vi "Terminate.vi"(8 "error in (no error)":errorcluster, 10 "Message in":refnum<class "TerminateMessage.lvclass">, 11 "DAQCascade512 in":refnum<class "DAQCascade512.lvclass">) -> (0 "error out":errorcluster, 3 "DAQCascade512 out":refnum<class "DAQCascade512.lvclass">)   [LabVIEW 2012, in "DAQCascade512.lvclass"]
doc: "This member function is called when the statemachine in the run.vi receives an 'terminate' command. It closes the RabbitMQ connection. \n\nOverride this member function in your derived class to release all previously acquired resources (but don't forget to call the parent method). If your component has subcomponents, they count as resources, and you have to release them by calling their own terminate functions."
uses:
  DAQCascade512.lvclass
  <vilib>/Distrio/Murmex/TerminateMessage/TerminateMessage.lvclass
  <vilib>/Distrio/Murmex/Murmex/Murmex.lvclass
  DAQCascade512.lvclass/DAQCascade512.ctl
panel:
  # "This method is called when the TERMINATE\ntrigger is sent. \n\nOverride this method when your component needs to\nrespond to this trigger. \n\nCall parent for proper implementation"
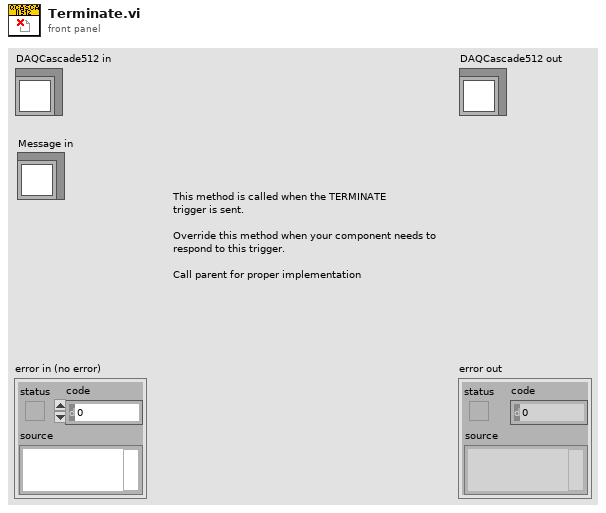
[diagram p1: front panel]
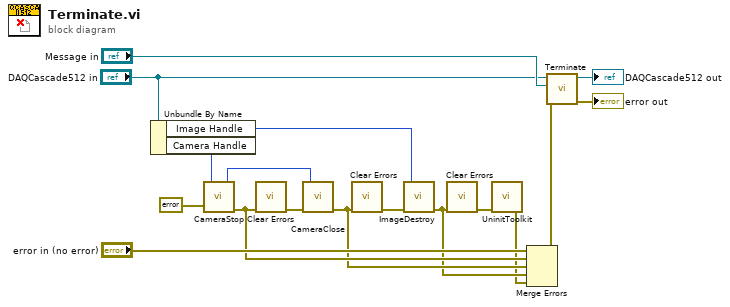
[diagram p0: block diagram]
diagram:
  n1 = Unbundle By Name("DAQCascade512 in") -> ("Image Handle"=w12:u32, "Camera Handle"=w13:u32)
  n2 = call <userlib>:"CameraStop.vi"("error in"=errorcluster {"status"=FALSE, "code"=0, "source"=""} ("error out"), "Camera Handle"=w13) -> ("error out"=w6:errorcluster, "Camera Handle"=w11:u32)
  n3 = call <vilib>:"Clear Errors.vi"("error in (no error)"=w6) -> ("error out"=w8:errorcluster)  [unwired: 6 in]
  n4 = call <userlib>:"CameraClose.vi"("error in"=w8, "Camera Handle"=w11) -> ("error out"=w5:errorcluster)
  n5 = call <vilib>:"Clear Errors.vi"("error in (no error)"=w5) -> ("error out"=w9:errorcluster)  [unwired: 6 in]
  n6 = call <userlib>:"ImageDestroy.vi"("error in"=w9, "Data handle"=w12) -> ("error out"=w4:errorcluster)
  n7 = call <vilib>:"Clear Errors.vi"("error in (no error)"=w4) -> ("error out"=w10:errorcluster)  [unwired: 6 in]
  n8 = call <userlib>:"UninitToolkit.vi"("error in"=w10) -> ("error out"=w3:errorcluster)
  n9 = Merge Errors("error in (no error)", w6, w5, w4, w3) -> (w2:errorcluster)
  n10 = call-parent "Terminate.vi"("error in (no error)"=w2, "Message in"="Message in", "Murmex in"="DAQCascade512 in") -> ("error out"=→"error out":errorcluster, "Murmex out"=→"DAQCascade512 out":refnum<class "DAQCascade512.lvclass">)  [unwired: 7 in]
